vi "Rapid_Scan_Trigs.vi"(0 "Board ID":u8=1 min=1 max=32 step=1, 1 "Program (1)":u8=4 format="%.0x", 2 "Start Position":i32=500000, 3 "BKPT Shift":i32, 5 "Scan Axis":u8=1 min=1 max=32 step=1, 7 "Pause?":bool, 9 "# frames/ s":sgl, 11 "error in (no error)":errorcluster, 12 "overshoot":i32=500, 13 "step interval":u32, 14 "Total Steps (one way)":i32) -> (4 "Bd ID Out":u8, 8 "Axis Resource out":u16(ring) items=["Axis Control"=0, "Axis 1"=1, "Axis 2"=2, "Axis 3"=3, "Axis 4"=4, "Axis 5"=5, "Axis 6"=6, "Axis 7"=7, "Axis 8"=8, "Vector Space Control"=16, "Vector Space 1"=17, "Vector Space 2"=18, "Vector Space 3"=19, "Vector Space 4"=20, "Encoder Control"=32, "Encoder 1"=33, "Encoder 2"=34, "Encoder 3"=35, "Encoder 4"=36, "Encoder 5"=37, "Encoder 6"=38, "Encoder 7"=39, "Encoder 8"=40, "DAC Channel 1"=49, "DAC Channel 2"=50, "DAC Channel 3"=51, "DAC Channel 4"=52, "DAC Channel 5"=53, "DAC Channel 6"=54, "DAC Channel 7"=55, "DAC Channel 8"=56, "Stepper Output 1"=65, "Stepper Output 2"=66, "Stepper Output 3"=67, "Stepper Output 4"=68, "Stepper Output 5"=69, "Stepper Output 6"=70, "Stepper Output 7"=71, "Stepper Output 8"=72, "ADC Channel 1"=81, "ADC Channel 2"=82, "ADC Channel 3"=83, "ADC Channel 4"=84, "ADC Channel 5"=85, "ADC Channel 6"=86, "ADC Channel 7"=87, "ADC Channel 8"=88], 10 "Program ID":u8 format="%.0x", 15 "error out":errorcluster)   [LabVIEW 2022 SP3]
doc: "EXAMPLE: DO_WHILE Loop (Onboard Programming Template)\n\nSUMMARY:\nThis FlexMotion example demonstrates the implementation of a DO_WHILE loop data structure in an onboard program. The C equivalent of the data structure implemented here is:\n\ndo {\n// code to be repeated\nloopVar = loopVar - increment;\n} while (loopVar != 0);\n\nTHEORY OF OPERATION:\nThe flow of the DO_WHILE loop data structure goes as follows:\n(1) Program storage is begun.\n(2) The DO_WHILE loop is set up. (Loop Variable and Increment are each defined and initialized.)\n(3) A code delimiter is set using label #1.\n(4) Code to be executed each time through loop is run (in the template program, the loop variable is decremented).\n(5) The loop variable or other test condition is checked.\n(6) If the test condition is true, then we jump back to label #1. Otherwise, the condition is false so the loop terminates.\n(7) Program storage is ended.\n\nDEVELOPMENT DETAILS:\nApplication Software: LabVIEW 5.0.x\nHardware: FlexMotion controller\nDriver Software: FlexMotion Software 4.0\n\nREQUIRED HARDWARE:\n(controller only)\n\nINSTRUCTIONS:\n(0) Initialize the FlexMotion controller before running this VI. \n(1) Add the FlexMotion functions you want to execute into the block diagram where noted.\n(2) Run the VI to store the program. (The program will not be executed at this time.)\n(3) You can then run the program you have stored by calling the run_prog.flx function with the appropriate program number.\n\nADDITIONAL NOTES:\n(a) You should read the following items before writing FlexMotion onboard programs:\n(1) The Onboard Programs section of the FlexMotion Hardware User Manual (page 4-9 in the November 1998 edition).\n(2) The section about onboard variables in your FlexMotion Software Reference Manual (pages 4-11 and 4-12 in the November 1998 edition)\n(3) You will find the chapter of the FlexMotion Software Reference Manual concerning the Onboard Programming functions to be an invaluable reference resource (Chapter 12 of the November 1998 edition) along with the online help for the VI functions.\n(b) This template repeats the DO_WHILE loop as long as an expression with a variable evaluates to be true. However, you may evaluate other conditions such as move complete status instead.\n\n*NOTE: This example is not supported on the 7334 controller."
uses:
  <vilib>/Motion/FlexMotion/FunctionsVIs/OnboardProgramming.llb/Jump to Label on Condition (8 axes).flx
  <vilib>/Motion/FlexMotion/FunctionsVIs/Trajectory.llb/Load Acceleration/Deceleration.flx
  <vilib>/Motion/FlexMotion/FunctionsVIs/MotionIO.llb/Set Inhibit MOMO (8 axes).flx
  <vilib>/Motion/FlexMotion/CustomControls/CustomControls.llb/Mask (8 axes).flx
  <vilib>/Motion/FlexMotion/FunctionsVIs/OnboardProgramming.llb/Wait on Condition (8 axes).flx
  <vilib>/Motion/FlexMotion/FunctionsVIs/OnboardProgramming.llb/Pause/Resume Program.flx
  <vilib>/Motion/FlexMotion/FunctionsVIs/StartStopMotion.llb/Start Motion (8 axes).flx
panel:
  out "acc (mm/s^2)":dbl
  out "velocity (mm/s)":dbl=10000.0
  out "1st BKPT":i32
  # "This will only work with735X controllers"
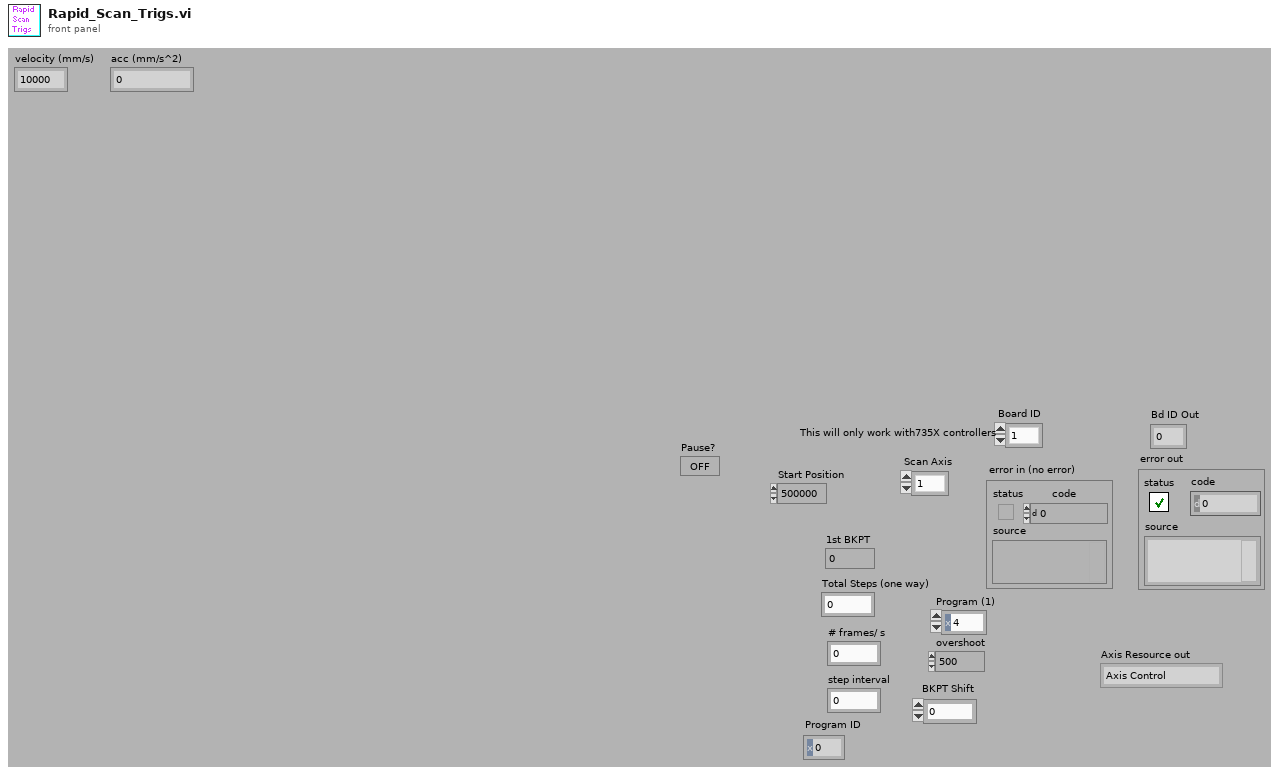
[diagram p1: front panel]
types:
  T1 = typedef "Var" = u8
  T2 = enum16{"Absolute Position", "Relative Position", "Velocity", "Relative to Cap Pos", "Modulus Position", "Absolute Contouring", "Relative Contouring"}
  T3 = enum16{"No Change", "Reset on Breakpoint", "Set on Breakpoint", "Toggle on Breakpoint", "Create Pulse on Breakpoint"}
  T4 = enum16{"Absolute Breakpoint", "Relative Breakpoint", "Modulo Breakpoint", "Periodic Breakpoint"}
  T5 = typedef "Mask (8 axes).flx" = cluster{"1":bool, "2":bool, "3":bool, "4":bool, "5":bool, "6":bool, "7":bool, "8":bool}
  T6 = typedef "Bd Id Out" = u8
  T7 = typedef "Resource Out (Enum).flx" = u16
  T8 = typedef "Resource Out.flx" = u8
  T9 = cluster{"0":bool, "1":bool, "2":bool, "3":bool, "4":bool, "5":bool, "6":bool, "7":bool, "8":bool}
  T10 = typedef "Condition Resource Out.flx" = u16
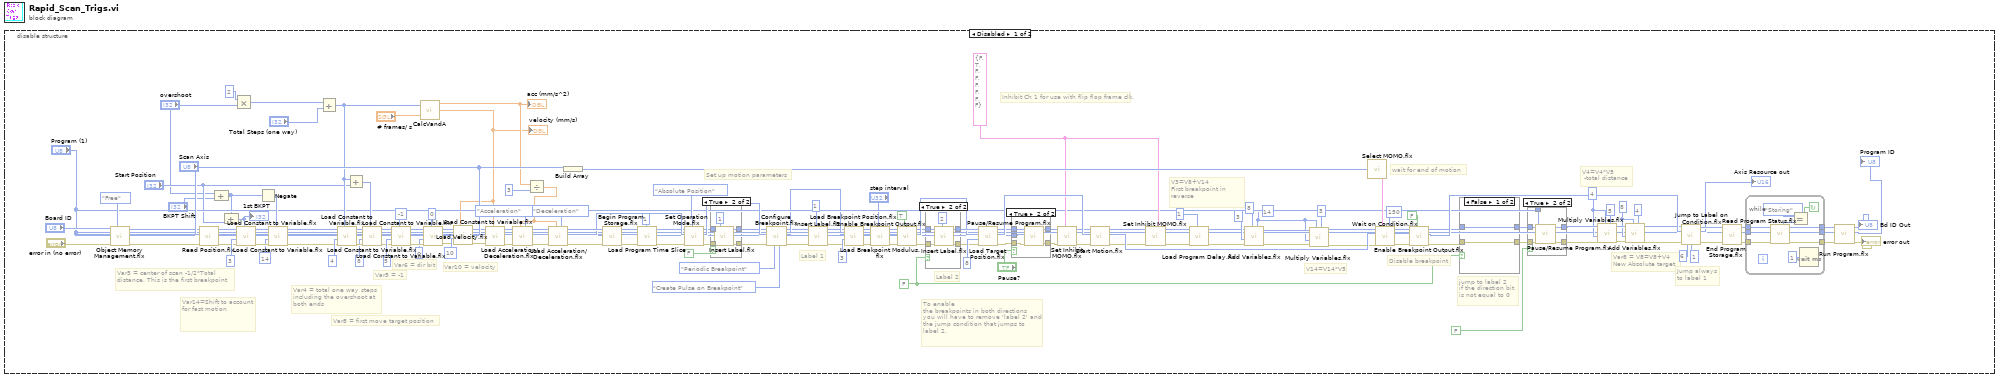
[diagram p0: block diagram]
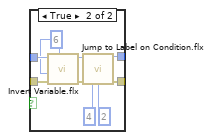
[diagram p6: hidden frame]
diagram:
  n1 = disable-structure shown="Disabled" {
    frame Disabled {
      w41 = 8
      w39 = 4
      w11 = 14
      w120 = FALSE ("Case Constant\n(See Context Help)")
      w82 = T5 {"1"=FALSE, "2"=TRUE, "3"=FALSE, "4"=FALSE, "5"=FALSE, "6"=FALSE, "7"=FALSE, "8"=FALSE} ("Must On (False)")
      # "V14=V14*V5"
      # "Var14=Shift to account for fast motion"
      # "Var10 = velocity"
      # "V3=V8+V14\nFirst breakpoint in reverse"
      # "Var6 = dir bit"
      # "Var8 = V8=V8+V4\nNew Absolute target"
      # "Var8 = first move target position"
      # "Inhibit Ch 1 for use with flip flop frame clk."
      # "Set up motion parameters"
      # "To enable\nthe breakpoints in both directions\nyou will have to remove 'label 2' and\nthe jump condition that jumps to \nlabel 2."
      # "Label 1"
      # "Label 2"
      # "jump to label 2\nif the direction bit\nis not equal to 0"
      # "Disable breakpoint"
      # "Jump always\nto label 1"
      # "V4=V4*V5\n -total distance"
      # "Var5 = -1"
      # "Var4 = total one way steps\nincluding the overshoot at \nboth ends"
      # "Var3 = center of scan -1/2*Total distance. This is the first breakpoint"
      # "wait for end of motion"
      n2 = call <vilib>:"Object Memory Management.flx"("Operation"=enum16{"Save", "Delete", "Free"}."Free" ("Operation (Free)"), "error in (no error)"="error in (no error)", "Object (1)"="Program (1)", "Board ID"="Board ID") -> ("error out"=w57:errorcluster, "Bd ID Out"=w58:T6)  [unwired: 4 out]
      n3 = call <vilib>:"Read Position.flx"("error in (no error)"=w57, "Axis"="Scan Axis", "Board ID"=w58) -> ("error out"=w123:errorcluster, "Bd ID Out"=w122:T6)  [unwired: 5 out]
      n4 = Compound Arithmetic op=ADD("overshoot", "BKPT Shift") -> (w14:i32)
      n5 = Compound Arithmetic op=ADD(w14, "Start Position") -> (w103:i32)
      "1st BKPT" <- w103
      n6 = Multiply(x=2, y="overshoot") -> (x*y=w136:i32)
      n7 = call <vilib>:"Load Constant to Variable.flx"("Value (0)"=w103, "error in (no error)"=w123, "Var"=3, "Board ID"=w122) -> ("error out"=w65:errorcluster, "Bd ID Out"=w66:T6)  [unwired: 4 out]
      n8 = Negate(x=w14) -> (-x=w62:i32)
      n9 = call <vilib>:"Load Constant to Variable.flx"("Value (0)"=w62, "error in (no error)"=w65, "Var"=14, "Board ID"=w66) -> ("error out"=w9:errorcluster, "Bd ID Out"=w10:T6)  [unwired: 4 out]
      n10 = Add(x=w136, y="Total Steps (one way)") -> (x+y=w61:i32)
      n11 = call <vilib>:"Load Constant to Variable.flx"("Value (0)"=w61, "error in (no error)"=w9, "Var"=4, "Board ID"=w10) -> ("error out"=w108:errorcluster, "Bd ID Out"=w109:T6)  [unwired: 4 out]
      n12 = Add(x=w61, y="Start Position") -> (x+y=w104:i32)
      n13 = call <vilib>:"Load Constant to Variable.flx"("Value (0)"=w104, "error in (no error)"=w108, "Var"=8, "Board ID"=w109) -> ("error out"=w107:errorcluster, "Bd ID Out"=w106:T6)  [unwired: 4 out]
      n14 = call <vilib>:"Load Constant to Variable.flx"("Value (0)"=-1, "error in (no error)"=w107, "Var"=5, "Board ID"=w106) -> ("error out"=w98:errorcluster, "Bd ID Out"=w99:T6)  [unwired: 4 out]
      n15 = call "CalcVandA.vi"("distance"=w61, "fps"="# frames/ s") -> ("Accel"=w59:dbl, "Velocity"=w6:dbl)  [unwired: 1 out]
      "velocity (mm/s)" <- w6
      "acc (mm/s^2)" <- w59
      n16 = call <vilib>:"Load Constant to Variable.flx"("Value (0)"=0, "error in (no error)"=w98, "Var"=6, "Board ID"=w99) -> ("error out"=w90:errorcluster, "Bd ID Out"=w91:T6)  [unwired: 4 out]
      n17 = call <vilib>:"Load Constant to Variable.flx"("Value (0)"=w6, "error in (no error)"=w90, "Var"=10, "Board ID"=w91) -> ("error out"=w89:errorcluster, "Bd ID Out"=w88:T6)  [unwired: 4 out]
      n18 = call <vilib>:"Load Velocity.flx"("Velocity (10000)"=w6, "error in (no error)"=w89, "Axis or Vector Space"="Scan Axis", "Board ID"=w88) -> ("error out"=w138:errorcluster, "Resource Output"=w139:T7, "Bd ID Out"=w140:T6)  [unwired: 3 out]
      n19 = Divide(x=w59, y=3) -> (x/y=w19:dbl)
      n20 = call "Load Acceleration/Deceleration.flx"("Acceleration Type (Both)"=enum16{"Both", "Acceleration", "Deceleration"}."Acceleration", "Acceleration (100000)"=w19, "error in (no error)"=w138, "Axis or Vector Space"=w139, "Board ID"=w140) -> ("error out"=w74:errorcluster, "Resource Output"=w70:T7, "Bd ID Out"=w75:T6)  [unwired: 2 out]
      n21 = call "Load Acceleration/Deceleration.flx"("Acceleration Type (Both)"=enum16{"Both", "Acceleration", "Deceleration"}."Deceleration", "Acceleration (100000)"=w19, "error in (no error)"=w74, "Axis or Vector Space"=w70, "Board ID"=w75) -> ("error out"=w73:errorcluster, "Resource Output"=w71:T7, "Bd ID Out"=w72:T6)  [unwired: 2 out]
      n22 = Build Array("Scan Axis") -> (w130:u8[])
      n23 = call <vilib>:"Begin Program Storage.flx"("error in (no error)"=w73, "Program (1)"="Program (1)", "Board ID"=w72) -> ("error out"=w55:errorcluster, "Resource Out"=w52:T8, "Bd ID Out"=w56:T6)  [unwired: 3 out]
      n24 = call <vilib>:"Load Program Time Slice.vi"("Time Slice (ms)"=u32 1, "error in (no error)"=w55, "Program"=w52, "Board ID"=w56) -> ("error out"=w54:errorcluster, "Bd ID Out"=w53:T6)  [unwired: 1 in, 2 out]
      n25 = call <vilib>:"Set Operation Mode.flx"("Position Mode (Absolute)"=T2."Absolute Position", "error in (no error)"=w54, "Axis or Vector Space"=w71, "Board ID"=w53) -> ("error out"=w116:errorcluster, "Resource Output"=w119:T7, "Bd ID Out"=w115:T6)  [unwired: 2 out]
      n26 = case shown="True" FALSE {
        tunnel: [w173 w177] -> w118
        tunnel: [w172 w176] -> w117
        tunnel: w116 -> [w172 w175]
        tunnel: w115 -> [w173 w174]
        frame False {
        }
        frame True {
          n27 = call <vilib>:"Insert Label.flx"("Label Number (1)"=1, "error in (no error)"=w175, "Board ID"=w174) -> ("error out"=w176:errorcluster, "Bd ID Out"=w177:T6)  [unwired: 4 out]
        }
      }
      n28 = call <vilib>:"Configure Breakpoint.flx"("Action (No Change)"=T3."Create Pulse on Breakpoint", "Mode (Absolute)"=T4."Periodic Breakpoint", "error in (no error)"=w117, "Axis or Encoder"=w119, "Board ID"=w118) -> ("error out"=w26:errorcluster, "Resource Output"=w28:T7, "Bd ID Out"=w27:T6)  [unwired: 1 in, 3 out]
      n29 = call <vilib>:"Insert Label.flx"("Label Number (1)"=1, "error in (no error)"=w26, "Board ID"=w27) -> ("error out"=w24:errorcluster, "Bd ID Out"=w25:T6)  [unwired: 4 out]
      n30 = call <vilib>:"Load Breakpoint Position.flx"("error in (no error)"=w24, "Inp Vect"=3, "Axis or Encoder"=w28, "Board ID"=w25) -> ("error out"=w34:errorcluster, "Resource Output"=w33:T7, "Bd ID Out"=w35:T6)  [unwired: 1 in, 2 out]
      n31 = call <vilib>:"Load Breakpoint Modulus.flx"("Breakpoint Modulus (0)"="step interval", "error in (no error)"=w34, "Axis or Encoder"=w33, "Board ID"=w35) -> ("error out"=w30:errorcluster, "Resource Output"=w32:T7, "Bd ID Out"=w31:T6)  [unwired: 3 out]
      n32 = call <vilib>:"Enable Breakpoint Output.flx"("Enable Breakpoint"=TRUE, "error in (no error)"=w30, "Axis or Encoder"=w32, "Board ID"=w31) -> ("error out"=w110:errorcluster, "Resource Output"=w112:T7, "Bd ID Out"=w111:T6)  [unwired: 3 out]
      n33 = case shown="True" w120 {
        tunnel: w111 -> [w180 w185]
        tunnel: w110 -> [w179 w184]
        tunnel: [w180 w183] -> w114
        tunnel: [w179 w182] -> w113
        frame False {
        }
        frame True {
          n34 = call <vilib>:"Insert Label.flx"("Label Number (1)"=2, "error in (no error)"=w184, "Board ID"=w185) -> ("error out"=w182:errorcluster, "Bd ID Out"=w183:T6)  [unwired: 4 out]
        }
      }
      n35 = call <vilib>:"Load Target Position.flx"("error in (no error)"=w113, "Inp Vect"=8, "Axis"=w112, "Board ID"=w114) -> ("error out"=w23:errorcluster, "Resource Output"=w83:T7, "Bd ID Out"=w20:T6)  [unwired: 1 in, 2 out]
      n36 = case shown="True" "Pause?" {
        tunnel: w23 -> [w158 w164]
        tunnel: w20 -> [w159 w163]
        tunnel: [w158 w162] -> w22
        tunnel: [w159 w161] -> w21
        tunnel: "Program (1)" -> [_ w160]
        frame False {
        }
        frame True {
          n37 = call "Pause/Resume Program.flx"("error in (no error)"=w164, "Program (1)"=w160, "Board ID"=w163) -> ("error out"=w162:errorcluster, "Bd ID Out"=w161:T6)  [unwired: 3 in, 1 out]
        }
      }
      n38 = call-poly <vilib>:"Set Inhibit MOMO.flx"("Must On (False)"=w82, "error in (no error)"=w22, "Board ID"=w21) -> ("error out"=w78:errorcluster, "Bd ID Out"=w79:T6)  [unwired: 1 in, 4 out]
      n39 = call-poly <vilib>:"Start Motion.flx"("error in (no error)"=w78, "Axis or Vector Space"=w83, "Board ID"=w79) -> ("error out"=w76:errorcluster, "Resource Output"=w80:T7, "Bd ID Out"=w77:T6)  [unwired: 1 in, 2 out]
      n40 = call-poly <vilib>:"Set Inhibit MOMO.flx"("Must Off (False)"=w82, "error in (no error)"=w76, "Board ID"=w77) -> ("error out"=w3:errorcluster, "Bd ID Out"=w47:T6)  [unwired: 1 in, 4 out]
      n41 = call <vilib>:"Load Program Delay.flx"("Delay Value (1 ms)"=u32 1, "error in (no error)"=w3, "Board ID"=w47) -> ("error out"=w2:errorcluster, "Bd ID Out"=w4:T6)  [unwired: 4 in]
      n42 = call <vilib>:"Add Variables.flx"("Var 2"=w11, "Var 1"=T1 8, "error in (no error)"=w2, "Ret Vect"=3, "Board ID"=w4) -> ("error out"=w17:errorcluster, "Bd ID Out"=w16:T6)  [unwired: 3 out]
      n43 = call <vilib>:"Multiply Variables.flx"("Var 2"=5, "Var 1"=w11, "error in (no error)"=w17, "Ret Vect"=w11, "Board ID"=w16) -> ("error out"=w8:errorcluster, "Bd ID Out"=w7:T6)  [unwired: 3 out]
      n44 = call <vilib>:"Select MOMO.flx"("Resource"=w130) -> ("Must On/Off"=w142:T9)
      n45 = call-poly <vilib>:"Wait on Condition.flx"("Board ID"=w7, "Must On (False)"=w142, "Timeout (1)"=150, "Resource (0)"=w80, "error in (no error)"=w8) -> ("Bd ID Out"=w101:T6, "Condition Resource Out"=w94:T10, "error out"=w102:errorcluster)  [unwired: 4 in, 4 out]
      n46 = call <vilib>:"Enable Breakpoint Output.flx"("Enable Breakpoint"=FALSE, "error in (no error)"=w102, "Axis or Encoder"=w94, "Board ID"=w101) -> ("error out"=w85:errorcluster, "Resource Output"=w93:T7, "Bd ID Out"=w86:T6)  [unwired: 3 out]
      n47 = case shown="False" w120 {
        tunnel: w85 -> [w186 w191]
        tunnel: w86 -> [w187 w192]
        tunnel: [w187 w194] -> w51
        tunnel: [w186 w193] -> w50
        frame False {
        }
        frame True {
          w188 = 6
          n48 = call <vilib>:"Invert Variable.flx"("Var 1"=w188, "error in (no error)"=w191, "Ret Vect"=w188, "Board ID"=w192) -> ("error out"=w190:errorcluster, "Bd ID Out"=w189:T6)  [unwired: 4 out]
          n49 = call-poly <vilib>:"Jump to Label on Condition.flx"("Board ID"=w189, "error in (no error)"=w190, "Condition Code (True)"=4, "Jump to Label (1)"=2) -> ("Bd ID Out"=w194:T6, "error out"=w193:errorcluster)  [unwired: 4 in, 6 out]
        }
      }
      n50 = case shown="True" FALSE {
        tunnel: w50 -> [w165 w171]
        tunnel: w51 -> [w166 w170]
        tunnel: [w165 w169] -> w45
        tunnel: [w166 w168] -> w46
        tunnel: "Program (1)" -> [_ w167]
        frame False {
        }
        frame True {
          n51 = call "Pause/Resume Program.flx"("error in (no error)"=w171, "Program (1)"=w167, "Board ID"=w170) -> ("error out"=w169:errorcluster, "Bd ID Out"=w168:T6)  [unwired: 3 in, 1 out]
        }
      }
      n52 = call <vilib>:"Multiply Variables.flx"("Var 2"=5, "Var 1"=w39, "error in (no error)"=w45, "Ret Vect"=w39, "Board ID"=w46) -> ("error out"=w42:errorcluster, "Bd ID Out"=w48:T6)  [unwired: 3 out]
      n53 = call <vilib>:"Add Variables.flx"("Var 2"=4, "Var 1"=w41, "error in (no error)"=w42, "Ret Vect"=w41, "Board ID"=w48) -> ("error out"=w43:errorcluster, "Bd ID Out"=w44:T6)  [unwired: 3 out]
      n54 = call-poly <vilib>:"Jump to Label on Condition.flx"("Board ID"=w44, "Resource (0)"=w93, "error in (no error)"=w43, "Condition Code (True)"=6, "Jump to Label (1)"=1) -> ("Bd ID Out"=w145:T6, "Condition Resource Out"=→"Axis Resource out":T10, "error out"=w144:errorcluster)  [unwired: 3 in, 5 out]
      n55 = call <vilib>:"End Program Storage.flx"("error in (no error)"=w144, "Program (1)"="Program (1)", "Board ID"=w145) -> ("error out"=w157:errorcluster, "Bd ID Out"=w156:T6)  [unwired: 4 out]
      n56 = while {
        tunnel: w156 -> [w206]
        tunnel: w157 -> [w205]
        tunnel: [w204] -> w152
        tunnel: [w203] -> w150
        tunnel: [w198] -> w151
        tunnel: "Program (1)" -> [w197]
        stop <- w200 continue-if-true
        n57 = call <vilib>:"Read Program Status.flx"("error in (no error)"=w205, "Program (1)"=w197, "Board Id"=w206) -> ("error out"=w203:errorcluster, "Resource Out"=w198:T8, "Bd Id Out"=w204:T6, "Program Status"=w201:enum16{"Done", "Playing", "Paused", "Storing"})  [unwired: 3 out]
        n58 = Equal?(x=enum16{"Done", "Playing", "Paused", "Storing"}."Storing" ("Program Status"), y=w201) -> (x = y?=w200:bool)
        n59 = Wait (ms)(milliseconds to wait=1) -> ()  [unwired: 1 out]
      }
      n60 = call <vilib>:"Run Program.flx"("error in (no error)"=w150, "Program (1)"=w151, "Board ID"=w152) -> ("error out"=→"error out":errorcluster, "Resource Out"=→"Program ID":T8, "Bd ID Out"=→"Bd ID Out":T6)  [unwired: 3 out]
    }
    frame Enabled {
    }
  }
